vi "SQL_Trigger_Bckup.vi"(8 "error in (no error)":errorcluster) -> (0 "error out":errorcluster)   [LabVIEW 2020]
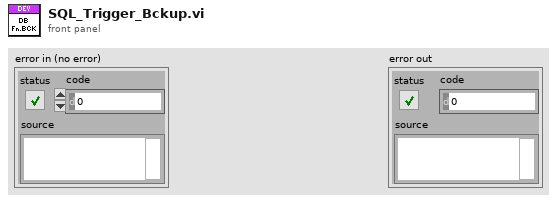
[diagram p1: front panel]
types:
  T1 = enum32{"invalid app kind", "Development System", "Run Time System", "Student Edition", "Embedded LabVIEW", "Evaluation", "Custom"}
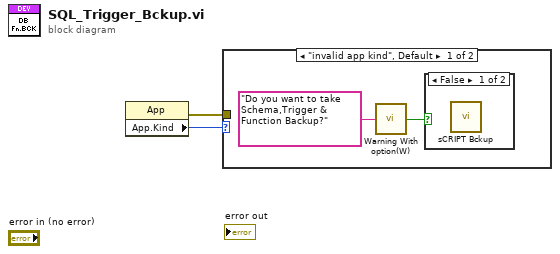
[diagram p0: block diagram]
diagram:
  n1 = property class="App"() -> (error out=w2:errorcluster, "App.Kind"=w1:T1)  [unwired: 2 in, 1 out]
  n2 = case shown="\"invalid app kind\", Default" w1 {
    tunnel: w2 -> [_ _]
    frame "invalid app kind", Default {
      n3 = call <userlib>:"Warning With option(W).vi"("Warning in"="Do you want to take Schema,Trigger & Function Backup?") -> ("Cancel ?"=w3:bool)  [unwired: 13 in, 1 out]
      n4 = case shown="False" w3 {
        frame False {
          n5 = call "sCRIPT Bckup.vi"() -> ()  [unwired: 12 in]
        }
        frame True {
        }
      }
    }
    frame "Run Time System" {
    }
  }
